vi "ShooterUnegaged.vi"(10 "Buttons":bool[](array[boolean]), 11 "Cluster":T1) -> ()   [LabVIEW 2015]
doc: "This code runs if the shooter is unengaged.\nIt checks the photo eye for blcoking and then checks if we are sucking in or out.s"
uses:
  constants/constants.ctl
  <vilib>/Rock Robotics/SystemInterfaces/DIO/FPGA_DIOPWMChannel.ctl
panel:
  # "ShooterMotors"
  # "DriveMotors- CAN Bus"
  # "PWM"
  # "ClimberMotors"
  # "CAN Bus"
  # "CAN Bus"
  # "PWM"
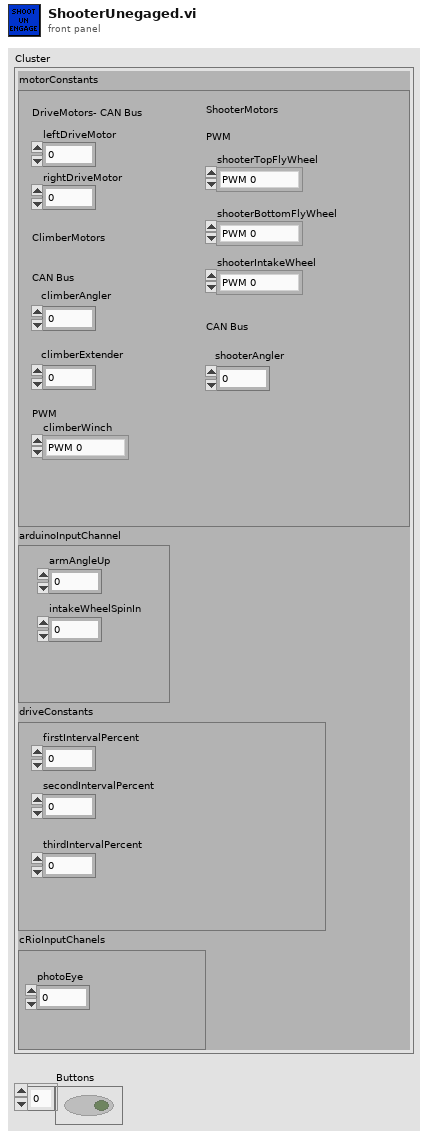
[diagram p1: front panel]
types:
  T1 = typedef "constants.ctl" = cluster{"motorConstants":cluster{"leftDriveMotor":i32, "rightDriveMotor":i32, "climberAngler":i32, "climberWinch":T2, "shooterTopFlyWheel":T2, "shooterBottomFlyWheel":T2, "climberExtender":i32, "shooterAngler":i32, "shooterIntakeWheel":T2}, "arduinoInputChannel":cluster{"armAngleUp":i32, "intakeWheelSpinIn":i32}, "driveConstants":cluster{"firstIntervalPercent":dbl, "secondIntervalPercent":dbl, "thirdIntervalPercent":dbl}, "cRioInputChanels":cluster{"photoEye":i32}}
  T2 = typedef "FPGA_DIOPWMChannel.ctl" = enum8{"PWM 0", "PWM 1", "PWM 2", "PWM 3", "PWM 4", "PWM 5", "PWM 6", "PWM 7", "PWM 8", "PWM 9", "PWM MXP 0", "PWM MXP 1", "PWM MXP 2", "PWM MXP 3", "PWM MXP 4", "PWM MXP 5", "PWM MXP 6", "PWM MXP 7", "PWM MXP 8", "PWM MXP 9", "Invalid"}
  T3 = typedef "WPI_DigitalInputDevRef.ctl" = cluster{"DevStatus":errorcluster, "DIO Channel":T4}
  T4 = typedef "FPGA_DIOChannel.ctl" = enum8{"DIO 0", "DIO 1", "DIO 2", "DIO 3", "DIO 4", "DIO 5", "DIO 6", "DIO 7", "DIO 8", "DIO 9", "DIO MXP 0", "DIO MXP 1", "DIO MXP 2", "DIO MXP 3", "DIO MXP 4", "DIO MXP 5", "DIO MXP 6", "DIO MXP 7", "DIO MXP 8", "DIO MXP 9", "DIO MXP 10", "DIO MXP 11", "DIO MXP 12", "DIO MXP 13", "DIO MXP 14", "DIO MXP 15", "Invalid"}
  T5 = typedef "WPI_MotorControlDeviceRef.ctl" = cluster{"DeviceStatus":errorcluster, "Type":T6, "PWM":cluster{"PWM Channel":T2, "DeadBand":T7}, "CAN":cluster{"Device Number":u8, "Control Mode":T8, "Semaphore":T9, "Max Vout":dbl, "TalonSRX Control Mode":T10}, "Invert":bool}
  T6 = typedef "WPI_MotorControlType.ctl" = enum16{"PWM", "CAN", "CANTalonSRX"}
  T7 = typedef "WPI_PWMDeadband.ctl" = cluster{"Name":string, "maxPositivePwm":i32, "minPositivePwm":i32, "centerPwm":i32, "maxNegativePwm":i32, "minNegativePwm":i32, "angularRange":u16}
  T8 = typedef "WPI_CANJaguar_ControlMode.ctl" = enum8{"Percent VBus", "Current", "Speed", "Position", "Voltage"}
  T9 = typedef "Semaphore RefNum" = refnum<k1>
  T10 = typedef "WPI_CANTalonSRX_APIControlMode.ctl" = enum8{"Percent VBus", "Speed", "Position", "Slave", "Unchanged / Invalid", "Voltage Compensation", "Current", "Motion Profile"}
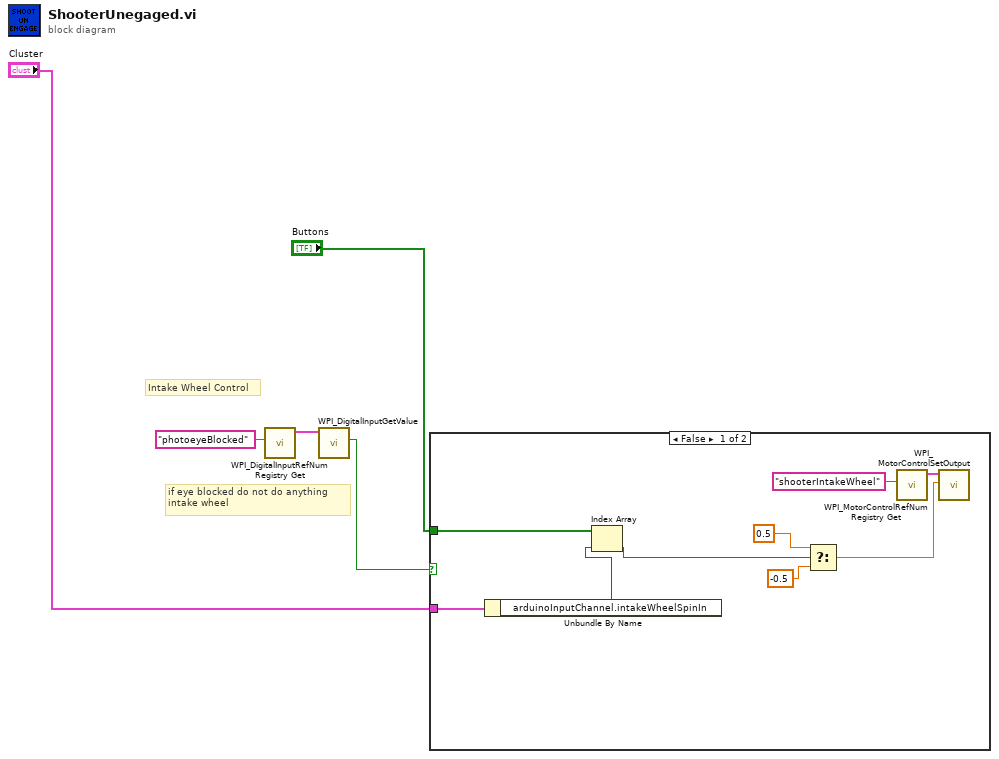
[diagram p0: block diagram]
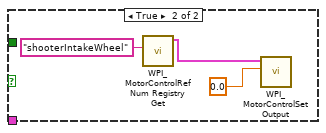
[diagram p2: hidden frame]
diagram:
  # "if eye blocked do not do anything \nintake wheel"
  # "Intake Wheel Control"
  n1 = call <vilib>:"WPI_DigitalInputRefNum Registry Get.vi"("refnum name"="photoeyeBlocked") -> ("DigitalInputDevRef"=w1:T3)  [unwired: 9 in, 1 out]
  n2 = call <vilib>:"WPI_DigitalInputGetValue.vi"("DigitalInputDevRef"=w1) -> ("Value"=w3:bool)  [unwired: 8 in, 2 out]
  n3 = case shown="False" w3 {
    tunnel: "Cluster" -> [w11 _]
    tunnel: "Buttons" -> [w10 _]
    frame False {
      n4 = Unbundle By Name(w11) -> ("arduinoInputChannel.intakeWheelSpinIn"=w12:i32)
      n5 = Index Array(array=w10, index=w12) -> (element=w9:bool)
      n6 = Select(t=0.5, s=w9, f=-0.5) -> (s? t:f=w6:dbl)
      n7 = call <vilib>:"WPI_MotorControlRefNum Registry Get.vi"("refnum name"="shooterIntakeWheel") -> ("MotorControlDevRef"=w13:T5)  [unwired: 9 in, 1 out]
      n8 = call <vilib>:"WPI_MotorControlSetOutput.vi"("Output"=w6, "MotorControlDevRef"=w13) -> ()  [unwired: 7 in, 3 out]
    }
    frame True {
      n9 = call <vilib>:"WPI_MotorControlRefNum Registry Get.vi"("refnum name"="shooterIntakeWheel") -> ("MotorControlDevRef"=w16:T5)  [unwired: 9 in, 1 out]
      n10 = call <vilib>:"WPI_MotorControlSetOutput.vi"("Output"=0.0, "MotorControlDevRef"=w16) -> ()  [unwired: 7 in, 3 out]
    }
  }
